vi "MainRunExp.vi"() -> ()   [LabVIEW 2019, in "MotorPID.lvlib"]
uses:
  MotorPID.lvlib
  RunState.ctl
  <vilib>/myRIO/Instrument Drivers/Onboard IO/DIO/typedefs/DIO Reference.ctl
  <vilib>/myRIO/Common/Instrument Driver Framework/Utilities/typedefs/myRIO Generic Hardware Reference.ctl
  <vilib>/myRIO/Common/Instrument Driver Framework/Utilities/typedefs/Hardware Version Enum.ctl
  <vilib>/myRIO/Common/Instrument Driver Framework/Utilities/typedefs/myRIO v1.0 Reference.ctl
  <vilib>/myRIO/Common/Instrument Driver Framework/Utilities/typedefs/Generic FPGA Reference.ctl
  <vilib>/myRIO/Common/Instrument Driver Framework/myRIO v1.0/DIO/typedefs/DIO Channels List.ctl
  <vilib>/myRIO/Common/Instrument Driver Framework/myRIO v1.0/DIO/typedefs/DIO Channels Enum.ctl
  <vilib>/userDefined/High Color/nirio_resource_hc.ctl
  <vilib>/Platform/TimedLoop/XDataNode/timing_clust.ctl
  <vilib>/Platform/TimedLoop/XDataNode/nitl_modes.ctl
  <vilib>/Platform/TimedLoop/XDataNode/wakeup.ctl
  <vilib>/myRIO/Common/Instrument Driver Framework/Utilities/vis/Is FPGA Ref Available.vi
  <vilib>/myRIO/Common/Instrument Driver Framework/ELVIS III v1.0/DIO/vis/ELVIS III v1.1 Open DIO.vi
  <vilib>/myRIO/Instrument Drivers/Onboard IO/DIO/vis/Write.vi
  <vilib>/myRIO/Common/Instrument Driver Framework/Utilities/vis/Validate Channels.vi
  <vilib>/myRIO/Common/Instrument Driver Framework/ELVIS III v1.0/DIO/vis/ELVIS III v1.0 Reserve DIO.vi
  <vilib>/myRIO/Common/Instrument Driver Framework/myRIO v1.0/UART/vis/myRIO v1.0 Close UART.vi
  <vilib>/myRIO/Common/Instrument Driver Framework/ELVIS III v1.0/DIO/vis/ELVIS III v1.0 Build MUX Configuration DIO.vi
  <vilib>/myRIO/Common/Instrument Driver Framework/ELVIS III v1.0/Resource Manager/vis/ELVIS III v1.0 Reserve Channel List.vi
  <vilib>/myRIO/Common/Instrument Driver Framework/ELVIS III v1.0/Resource Manager/vis/ELVIS III v1.0 Create Configuration List.vi
  <vilib>/myRIO/Common/Instrument Driver Framework/ELVIS III v1.0/Resource Manager/vis/ELVIS III v1.0 Reserve Channel.vi
  <vilib>/myRIO/Common/Instrument Driver Framework/ELVIS III v1.0/Resource Manager/vis/ELVIS III v1.0 Unreserve Channel.vi
  <vilib>/myRIO/Common/Instrument Driver Framework/ELVIS III v1.0/Resource Manager/vis/ELVIS III v1.0 Build Mutex Name.vi
  <vilib>/Utility/VariantDataType/GetNumericInfo.vi
  <vilib>/Utility/error.llb/Error Cluster From Error Code.vi
  <vilib>/myRIO/Common/Instrument Driver Framework/ELVIS III v1.0/ELVIS III v1.1 Open.vi
  <vilib>/myRIO/Common/Instrument Driver Framework/Utilities/vis/IO Manager.vi
  <vilib>/myRIO/Common/Instrument Driver Framework/Utilities/vis/Configuration Manager.vi
  <vilib>/myRIO/Common/Instrument Driver Framework/ELVIS III v1.0/Resource Manager/vis/ELVIS III v1.0 Configure IO.vi
  <vilib>/myRIO/Common/Instrument Driver Framework/myRIO v1.0/myRIO v1.0 Close.vi
  <vilib>/myRIO/Common/Instrument Driver Framework/ELVIS III v1.0/DIO/vis/ELVIS III v1.0 Write DIO.vi
  <vilib>/addons/control/pid/pid.llb/PID (DBL).vi
  <vilib>/myRIO/Common/Instrument Driver Framework/Utilities/vis/FPGA Ref Manager.vi
  <vilib>/myRIO/Common/Instrument Driver Framework/ELVIS III v1.0/ELVIS III v1.0 Reset FPGA.vi
  <vilib>/myRIO/Common/Instrument Driver Framework/myRIO v1.0/IRQ/vis/myRIO v1.0 IRQ Info FGV.vi
  <vilib>/myRIO/Common/Instrument Driver Framework/myRIO v1.0/IRQ/vis/myRIO v1.0 Timer IRQ Info FGV.vi
  <vilib>/myRIO/Common/Instrument Driver Framework/myRIO v1.0/IRQ/vis/myRIO v1.0 ISR Agent.vi
  <vilib>/myRIO/Instrument Drivers/Utilities/vis/Reset Index.vi
  <vilib>/myRIO/Common/Instrument Driver Framework/myRIO v1.0/Resource Manager/vis/myRIO v1.0 Block Write Resource Manager.vi
  <vilib>/myRIO/Express VI/Onboard IO/DO/DO Express VI.xnode
  <vilib>/myRIO/Instrument Drivers/Onboard IO/DIO/vis/myRIO DIO Open.xnode
  <vilib>/Platform/TimedLoop/XDataNode/XDataNode.xnode
  <vilib>/Platform/TimedLoop/XDataNode/XDNodeRunTimeDep.lvlib
  <vilib>/myRIO/Instrument Drivers/Onboard IO/DIO/DIO.lvlib
  <vilib>/myRIO/Instrument Drivers/Utilities/Utilities.lvlib
  <vilib>/ptbypt/NI_PtbyPt.lvlib
  <vilib>/addons/control/pid/NI_PID_pid.lvlib
panel:
  out "x >= y?":bool
  out "Boolean":bool
  out "State":u16(ring) items=["StickReset", "MotorReset", "MotorHome", "RunUp", "Runing", "Exit"]
  out "Waveform Chart":T1(graph)
  in  "Setpoint(deg)":dbl(knob) scale=80.0..-80.0
  out "error out":errorcluster
  out "Position(deg)":dbl(knob) scale=80.0..-80.0
  in  "Reset":bool
  in  "Stop Button":bool
  out "MotorResetPOS":dbl[](array[numeric])
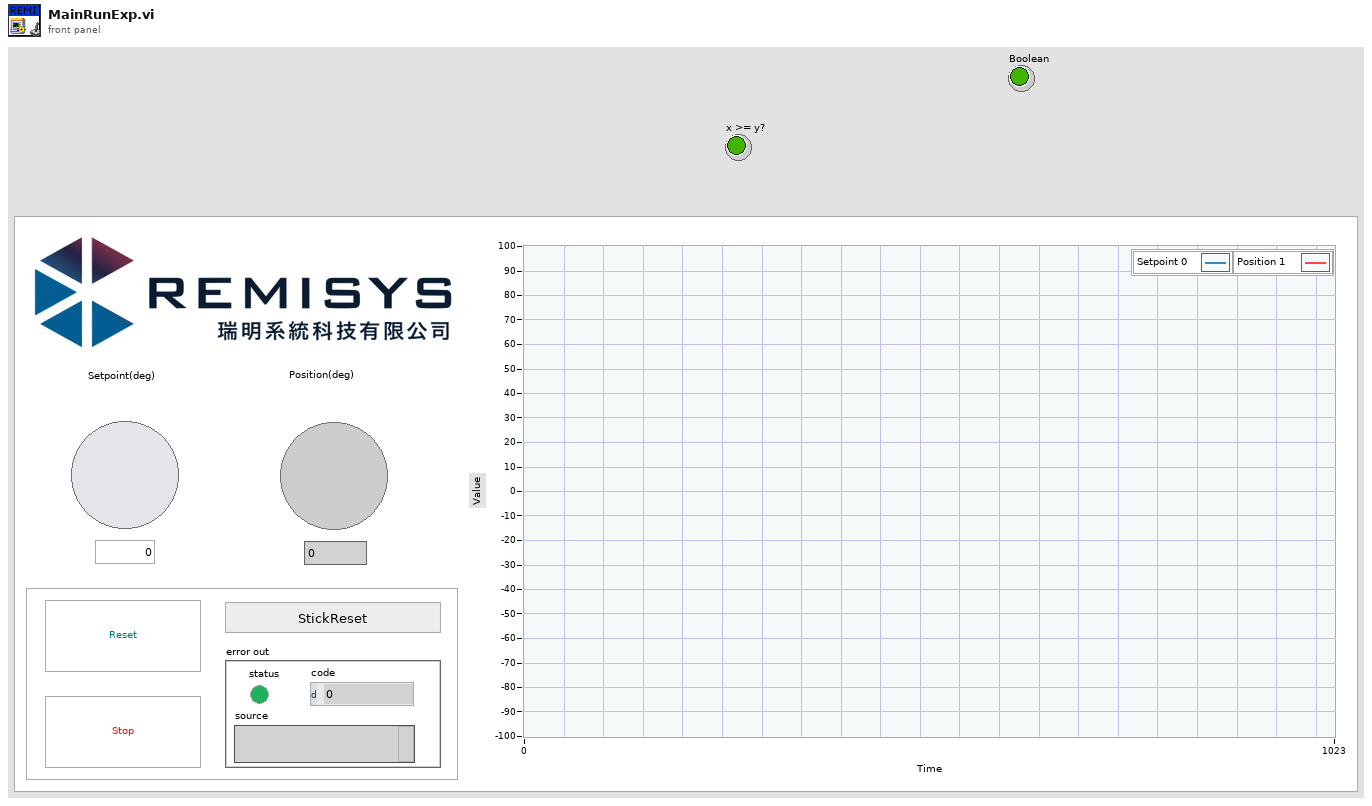
[diagram p1: front panel]
types:
  T1 = cluster{"Setpoint(deg)":dbl, "PresentPOS(deg)":dbl}
  T2 = typedef "MotorPID.lvlib/RunState.ctl" = enum16{"StickReset", "MotorReset", "MotorHome", "RunUp", "Runing", "Exit"}
  T3 = typedef "DIO.lvlib/DIO Reference.ctl" = cluster{"myRIO Reference":T4, "DIO Channels List":T8}
  T4 = typedef "myRIO Generic Hardware Reference.ctl" = cluster{"myRIO Model":T5, "myRIO Hardware Reference":T6}
  T5 = typedef "Hardware Version Enum.ctl" = enum16{"Unknown", "myRIO-1900", "myRIO-1950", "roboRIO", "NI ELVIS RIO CM", "ELVIS III"}
  T6 = typedef "myRIO v1.0 Reference.ctl" = cluster{"Generic FPGA Reference":T7, "Allow multiple opens":bool}
  T7 = typedef "Generic FPGA Reference.ctl" = refnum<k20>
  T8 = typedef "DIO Channels List.ctl" = T9[]
  T9 = typedef "DIO Channels Enum.ctl" = enum16{"Not Connected", "C/DIO0", "C/DIO1", "C/DIO2", "C/DIO3", "C/DIO4", "C/DIO5", "C/DIO6", "C/DIO7", "A/DIO0", "A/DIO1", "A/DIO2", "A/DIO3", "A/DIO4", "A/DIO5", "A/DIO6", "A/DIO7", "A/DIO8", "A/DIO9", "A/DIO10", "A/DIO11", "A/DIO12", "A/DIO13", "A/DIO14", "A/DIO15", "A/DIO16", "A/DIO17", "A/DIO18", "A/DIO19", "B/DIO0", "B/DIO1", "B/DIO2", "B/DIO3", "B/DIO4", "B/DIO5", "B/DIO6", "B/DIO7", "B/DIO8", "B/DIO9", "B/DIO10", "B/DIO11", "B/DIO12", "B/DIO13", "B/DIO14", "B/DIO15", "B/DIO16", "B/DIO17", "B/DIO18", "B/DIO19", "LED0", "LED1", "LED2", "LED3", "Button0", "DIO/DIO0", "DIO/DIO1", "DIO/DIO2", "DIO/DIO3", "DIO/DIO4", "DIO/DIO5", "DIO/DIO6", "DIO/DIO7", "DIO/DIO8", "DIO/DIO9", "SPI/CS0", "SPI/CS1", "SPI/CS2", "SPI/CS3", "LED RADIO (Green)", "LED RADIO (Red)", "LED COMM (Green)", "LED COMM (Red)", "LED MODE (Green)", "LED MODE (Red)"}
  T10 = typedef "nirio_resource_hc.ctl" = tag
  T11 = typedef "XDNodeRunTimeDep.lvlib/timing_clust.ctl" = cluster{"Expected End [f-1]":u64, "Actual End [f-1]":u64, "Finished Late? [f-1]":bool, "Expected End [i-1]":u64, "Actual End [i-1]":u64, "Finished Late? [i-1]":bool, "Expected Start [i]":u64, "Actual Start [i]":u64, "Expected Start [f]":u64, "Actual Start [f]":u64, "Source Name":string, "Structure Name":string, "Period":i64, "Deadline":i64, "Offset":i64, "Start":i64, "Priority":i32, "Timeout":i32, "Mode":T12, "Wakeup Reason":T13, "Error":errorcluster, "Source Type":string, "Secondary Source Type":string, "Global End Time":u64, "Global Start Time":u64, "Frame Duration":u64, "Iteration Duration":u64, "Assigned CPU":i32, "I/O Scan Engine Mode":u32}
  T12 = typedef "XDNodeRunTimeDep.lvlib/nitl_modes.ctl" = enum32{"No Change", "Process missed periods, maintain original phase", "Discard missed periods, maintain original phase", "Process missed periods, ignore original phase", "Discard missed periods, ignore original phase"}
  T13 = typedef "XDNodeRunTimeDep.lvlib/wakeup.ctl" = enum32{"Normal", "Aborted", "Asynchronous wakeup", "Timing source error", "Timed loop error", "Timeout"}
  T14 = cluster{"proportional gain (Kc)":dbl, "integral time (Ti, min)":dbl, "derivative time (Td, min)":dbl}
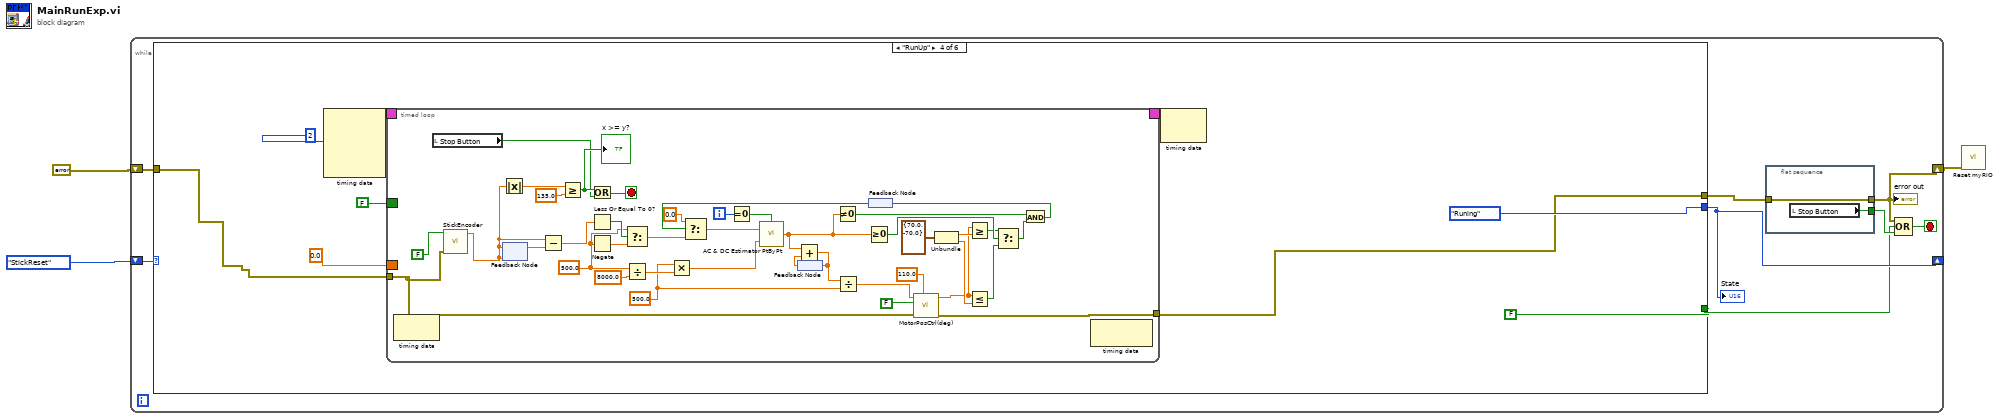
[diagram p0: block diagram]
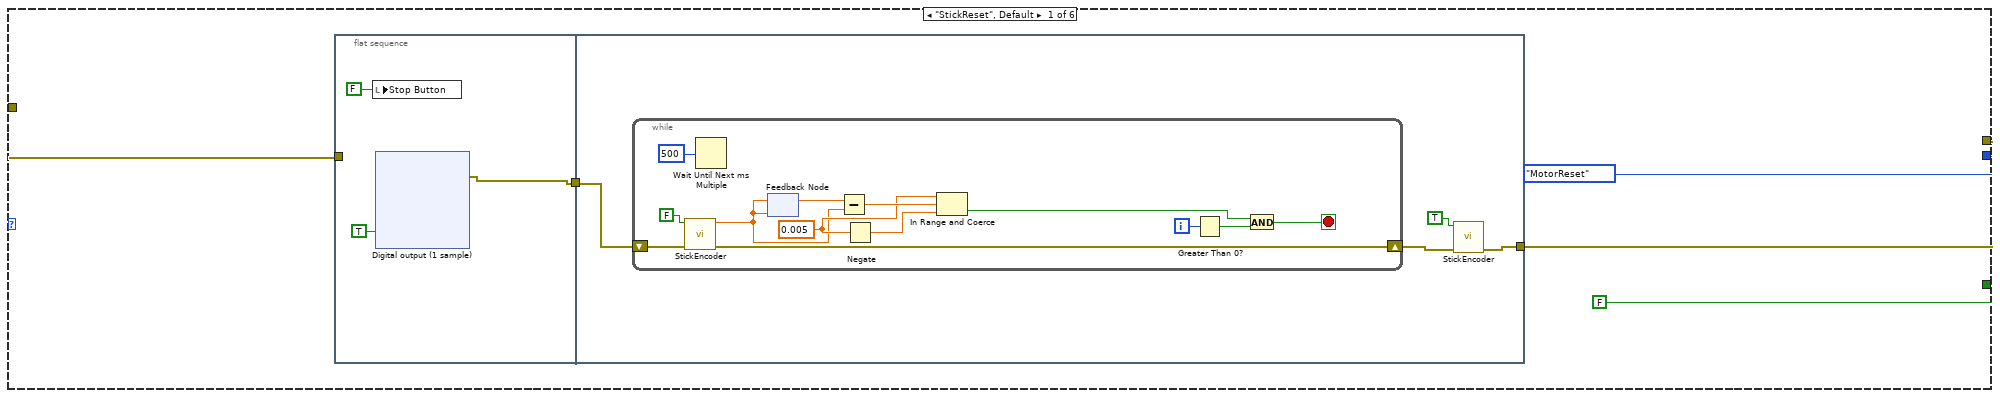
[diagram p2: hidden frame]
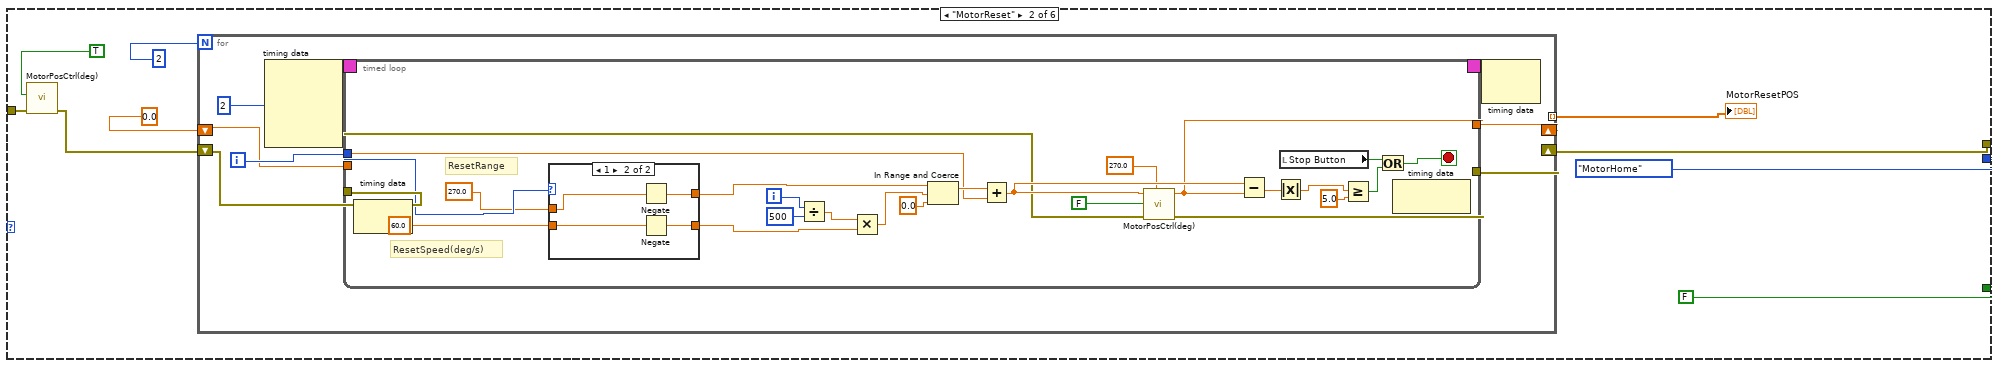
[diagram p3: hidden frame]
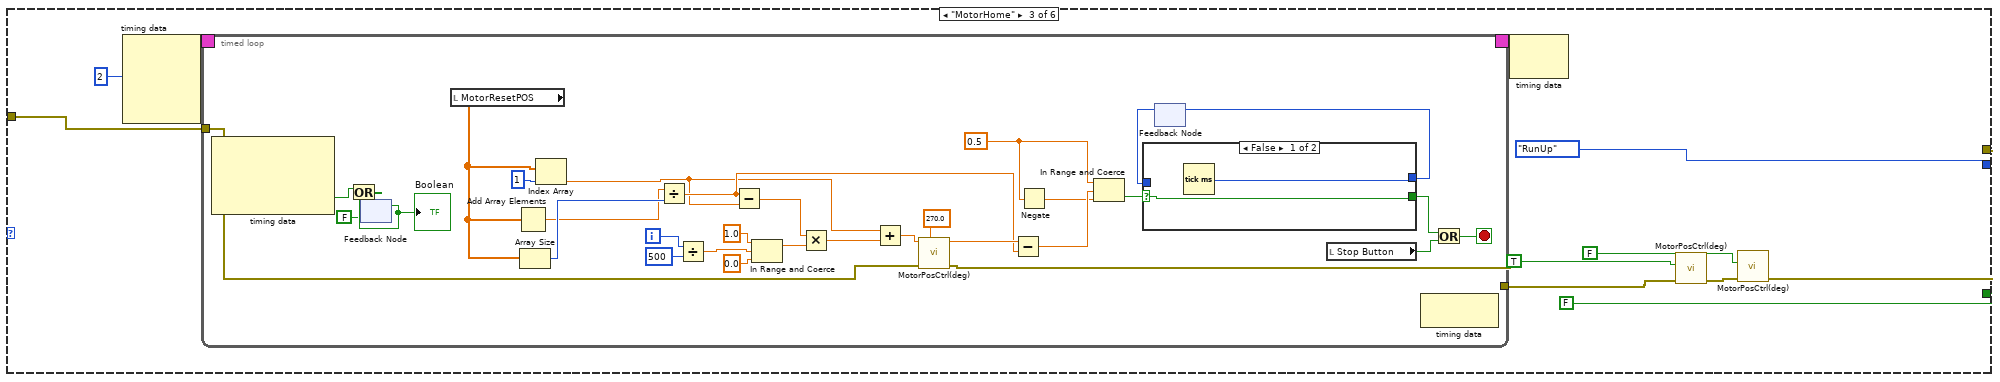
[diagram p5: hidden frame]
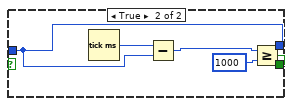
[diagram p6: hidden frame]
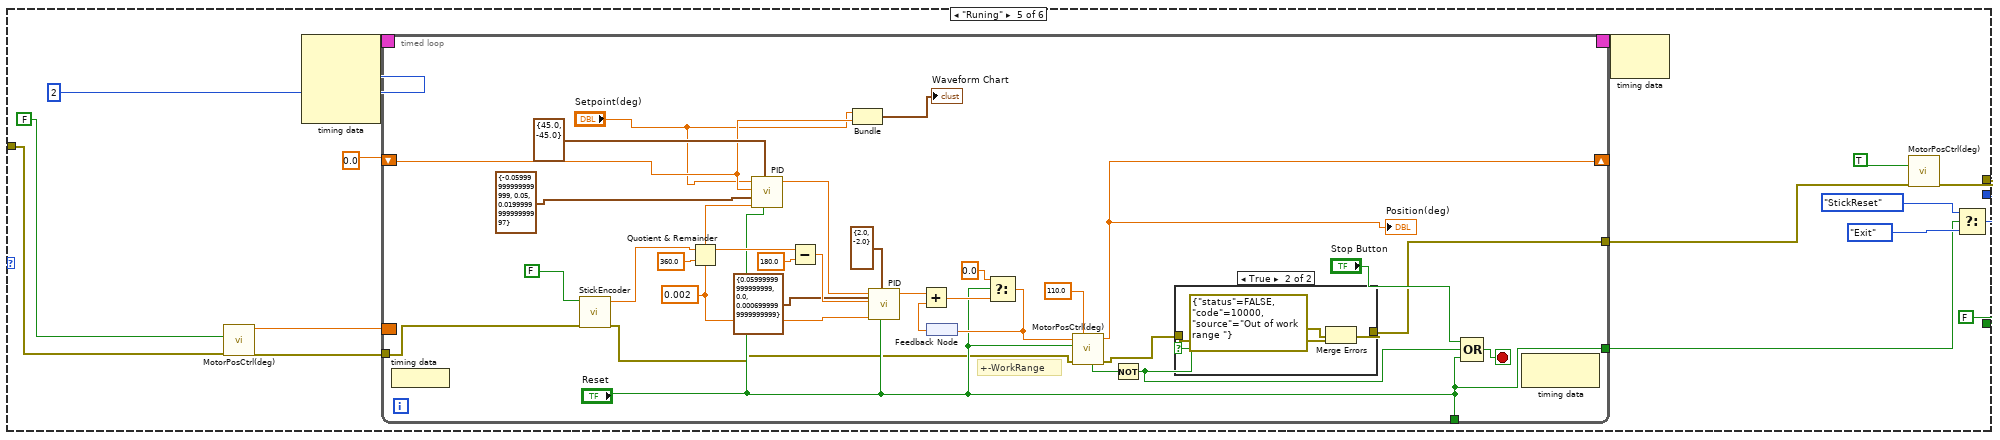
[diagram p7: hidden frame]
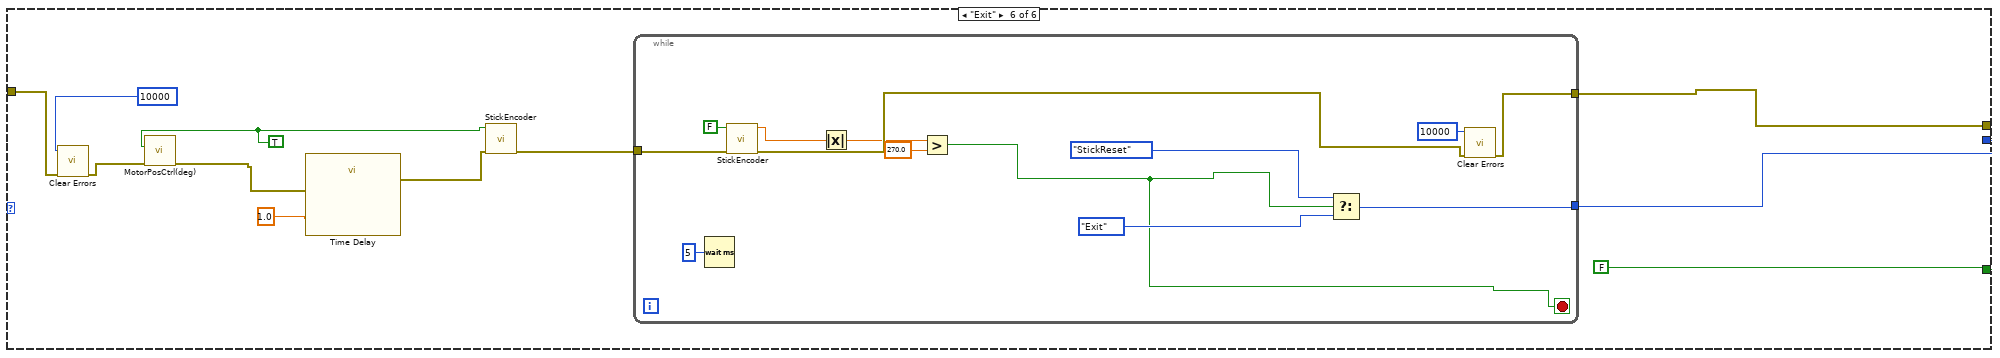
[diagram p9: hidden frame]
diagram:
  n1 = while {
    shift-right: [w6] -> _
    shift-left: RunState."StickReset" -> [w11]
    shift-right: [w5] -> w1
    shift-left: errorcluster {"status"=FALSE, "code"=0, "source"=""} ("error in (no error)") -> [w10]
    stop <- w9 stop-if-true
    n2 = case shown="\"RunUp\"" w11 {
      tunnel: w10 -> [w16 w76 w134 w185 w254 w303]
      tunnel: [w17 w82 w128 w184 w251 w301] -> w8
      tunnel: [RunState."MotorReset" RunState."MotorHome" RunState."RunUp" RunState."Runing" w248 w305] -> w6
      tunnel: [FALSE FALSE FALSE FALSE FALSE FALSE] -> w4
      frame "StickReset", Default {
        n3 = flat-sequence {
          tunnel: w16 -> [_]
          tunnel: [w19] -> w15
          tunnel: [w58] -> w17
          tunnel: w15 -> [w57]
          frame #0 {
            n4 = local write "Stop Button"(FALSE ("Stop Button")) -> ()
            n5 = xnode "Digital output (1 sample)"("ENA (A/DIO5)"=TRUE) -> ("error out"=w19:errorcluster)  [unwired: 1 in]
          }
          frame #1 {
            n6 = while {
              shift-right: [w73] -> w60
              shift-left: w57 -> [w72]
              i -> [w66]
              stop <- w63 stop-if-true
              w68 = 0.005 ("upper limit")
              n7 = call "StickEncoder.vi"("error in (no error)"=w72, "Reset Counter"=FALSE) -> ("error out"=w73:errorcluster, "PresentPOS(deg)"=w61:dbl)  [unwired: 8 in]
              n8 = Wait Until Next ms Multiple(millisecond multiple=u32 500) -> ()  [unwired: 1 out]
              n9 = feedback-in #1(w61) -> ()
              n10 = feedback #1(w61) -> (w70:dbl)
              n11 = Subtract(x=w70, y=w61) -> (x-y=w69:dbl)
              n12 = Negate(x=w68) -> (-x=w67:dbl)
              n13 = In Range and Coerce(upper limit=w68, x=w69, lower limit=w67) -> (In Range?=w65:bool)  [unwired: 1 out]
              n14 = Greater Than 0?(x=w66) -> (x > 0?=w64:bool)
              n15 = And(x=w65, y=w64) -> (x .and. y?=w63:bool)
            }
            n16 = call "StickEncoder.vi"("error in (no error)"=w60, "Reset Counter"=TRUE) -> ("error out"=w58:errorcluster)  [unwired: 8 in, 1 out]
          }
        }
      }
      frame "MotorReset" {
        n17 = call "MotorPosCtrl(deg).vi"("error in (no error)"=w76, "Reset Button"=TRUE) -> ("error out"=w77:errorcluster)  [unwired: 6 in, 3 out]
        n18 = for {
          N: 2 -> [_]
          shift-right: [w87] -> w82
          shift-left: w77 -> [w86]
          shift-right: [w83] -> _
          shift-left: 0.0 ("PresentPOS(deg)") -> [w84]
          tunnel: [w83] -> w79 mode=indexing
          i -> [w85]
          n19 = node-c288(i64 2 ("Period")) -> (w90:T11)  [unwired: 3 in]
          n20 = timed-loop {
            timing: w90 -> [_]
            timing-out: [_] -> w89
            tunnel: w86 -> [w91]
            tunnel: [w114] -> w87
            tunnel: w85 -> [w109]
            tunnel: [w97] -> w83
            tunnel: w84 -> [w106]
            i -> [w113]
            stop <- w101 stop-if-true
            # "ResetRange"
            # "ResetSpeed(deg/s)"
            n21 = node-c288() -> ()  [unwired: 1 in, 1 out]
            n22 = case shown="1" w109 {
              tunnel: [w116 w119] -> w108
              tunnel: [w115 w117] -> w104
              tunnel: 270.0 ("Target(deg)") -> [w116 w120]
              tunnel: 60.0 ("y") -> [w115 w118]
              frame 0, Default {
              }
              frame 1 {
                n23 = Negate(x=w120) -> (-x=w119:dbl)
                n24 = Negate(x=w118) -> (-x=w117:dbl)
              }
            }
            n25 = Divide(x=w113, y=500) -> (x/y=w112:dbl)
            n26 = Multiply(x=w112, y=w104) -> (x*y=w111:dbl)
            n27 = In Range and Coerce(upper limit=w108, x=w111, lower limit=0.0) -> (coerced(x)=w107:dbl)  [unwired: 1 out]
            n28 = Add(x=w107, y=w106) -> (x+y=w98:dbl)
            n29 = call "MotorPosCtrl(deg).vi"("WorkRange 2"=270.0 ("WorkRange"), "error in (no error)"=w91, "Reset Button"=FALSE, "Target(deg)"=w98) -> ("error out"=w114:errorcluster, "PresentPOS(deg)"=w97:dbl)  [unwired: 4 in, 2 out]
            n30 = Subtract(x=w98, y=w97) -> (x-y=w95:dbl)
            n31 = Absolute Value(x=w95) -> (abs(x)=w94:dbl)
            n32 = local read "Stop Button"() -> (w100:bool)
            n33 = Greater Or Equal?(x=w94, y=5.0) -> (x >= y?=w93:bool)
            n34 = Or(x=w100, y=w93) -> (x .or. y?=w101:bool)
            n35 = node-c288() -> ()  [unwired: 1 in, 1 out]
          }
          n36 = node-c288(w89) -> ()  [unwired: 1 out]
        }
        "MotorResetPOS" <- w79
      }
      frame "MotorHome" {
        n37 = node-c288(i64 2 ("Period")) -> (w136:T11)  [unwired: 3 in]
        n38 = timed-loop {
          timing: w136 -> [_]
          timing-out: [_] -> w135
          tunnel: w134 -> [w169]
          tunnel: [w163] -> w132
          i -> [w157]
          stop <- w143 stop-if-true
          w165 = 0.5
          n39 = node-c288() -> (w141:bool)  [unwired: 1 in, 3 out]
          n40 = feedback #2(FALSE) -> (w139:bool)
          "Boolean" <- w139
          n41 = Or(x=w141, y=w139) -> (x .or. y?=w140:bool)
          n42 = feedback-in #2(w140) -> ()
          n43 = local read "MotorResetPOS"() -> (w152:dbl[])
          n44 = Add Array Elements(numeric array=w152) -> (sum=w151:dbl)
          n45 = Array Size(array=w152) -> (size(s)=w168:i32)
          n46 = Index Array(array=w152, index=1) -> (element=w146:dbl)
          n47 = Divide(x=w151, y=w168) -> (x/y=w148:dbl)
          n48 = Divide(x=w157, y=500) -> (x/y=w155:dbl)
          n49 = Subtract(x=w148, y=w146) -> (x-y=w147:dbl)
          n50 = In Range and Coerce(upper limit=1.0, x=w155, lower limit=0.0) -> (coerced(x)=w150:dbl)  [unwired: 1 out]
          n51 = Multiply(x=w147, y=w150) -> (x*y=w149:dbl)
          n52 = Add(x=w146, y=w149) -> (x+y=w145:dbl)
          n53 = call "MotorPosCtrl(deg).vi"("WorkRange 2"=270.0 ("WorkRange"), "error in (no error)"=w169, "Target(deg)"=w145) -> ("error out"=w163:errorcluster, "PresentPOS(deg)"=w167:dbl)  [unwired: 5 in, 2 out]
          n54 = Subtract(x=w167, y=w148) -> (x-y=w166:dbl)
          n55 = Negate(x=w165) -> (-x=w164:dbl)
          n56 = In Range and Coerce(upper limit=w165, x=w166, lower limit=w164) -> (In Range?=w158:bool)  [unwired: 1 out]
          n57 = feedback #3() -> (w161:u32)  [unwired: 1 in]
          n58 = case shown="False" w158 {
            selector: w158 -> [w170 _]
            tunnel: [w171 w172] -> w162
            tunnel: w161 -> [_ w172]
            tunnel: [w170 w173] -> w159
            frame False {
              n59 = Tick Count (ms)() -> (millisecond timer value=w171:u32)
            }
            frame True {
              n60 = Tick Count (ms)() -> (millisecond timer value=w176:u32)
              n61 = Subtract(x=w176, y=w172) -> (x-y=w175:u32)
              n62 = Greater Or Equal?(x=w175, y=u32 1000) -> (x >= y?=w173:bool)
            }
          }
          n63 = feedback-in #3(w162) -> ()
          n64 = local read "Stop Button"() -> (w160:bool)
          n65 = node-c288() -> ()  [unwired: 1 in, 1 out]
          n66 = Or(x=w159, y=w160) -> (x .or. y?=w143:bool)
        }
        n67 = node-c288(w135) -> ()  [unwired: 1 out]
        n68 = call "MotorPosCtrl(deg).vi"("error in (no error)"=w132, "Reset Button"=TRUE) -> ("error out"=w129:errorcluster)  [unwired: 6 in, 3 out]
        n69 = call "MotorPosCtrl(deg).vi"("error in (no error)"=w129, "Reset Button"=FALSE) -> ("error out"=w128:errorcluster)  [unwired: 6 in, 3 out]
      }
      frame "RunUp" {
        n70 = node-c288(i64 2 ("Period")) -> (w190:T11)  [unwired: 3 in]
        n71 = timed-loop {
          timing: w190 -> [_]
          timing-out: [_] -> w189
          tunnel: w185 -> [w198]
          tunnel: [w193] -> w184
          border: 0.0 ("PresentPOS(deg)") -> [_]
          border: FALSE -> [_]
          i -> [w232]
          stop <- w226 stop-if-true
          w222 = 500.0 ("MaxSpeed(deg/s)")
          w212 = 500.0 ("x")
          n72 = node-c288() -> ()  [unwired: 1 in, 1 out]
          n73 = local read "Stop Button"() -> (w199:bool)
          n74 = call "StickEncoder.vi"("error in (no error)"=w198, "Reset Counter"=FALSE) -> ("PresentPOS(deg)"=w201:dbl)  [unwired: 8 in, 1 out]
          n75 = Absolute Value(x=w201) -> (abs(x)=w229:dbl)
          n76 = feedback-in #4(w201) -> ()
          n77 = feedback #4(w201) -> (w230:dbl)
          n78 = Subtract(x=w201, y=w230) -> (x-y=w225:dbl)
          n79 = Greater Or Equal?(x=w229, y=135.0) -> (x >= y?=w227:bool)
          "x >= y?" <- w227
          n80 = Or(x=w227, y=w199) -> (x .or. y?=w226:bool)
          n81 = Less Or Equal To 0?(x=w225) -> (x <= 0?=w224:bool)
          n82 = Negate(x=w222) -> (-x=w223:dbl)
          n83 = Select(t=w222, s=w224, f=w223) -> (s? t:f=w216:dbl)
          n84 = Divide(x=w222, y=8000.0 ("Acc(deg/ss)")) -> (x/y=w221:dbl)
          n85 = Multiply(x=w212, y=w221) -> (x*y=w202:dbl)
          n86 = Equal To 0?(x=w232) -> (x = 0?=w231:bool)
          n87 = feedback #5() -> (w219:dbl)
          n88 = feedback #6() -> (w217:bool)
          n89 = Select(t=0.0, s=w217, f=w216) -> (s? t:f=w214:dbl)
          n90 = call <vilib>:"AC & DC Estimator PtByPt.vi"("signal"=w214, "sample length"=w202, "initialize"=w231) -> ("DC estimate (V)"=w206:dbl)  [unwired: 2 out]
          n91 = Add(x=w206, y=w219) -> (x+y=w213:dbl)
          n92 = feedback-in #5(w213) -> ()
          n93 = Not Equal To 0?(x=w206) -> (x != 0?=w205:bool)
          n94 = Divide(x=w213, y=w212) -> (x/y=w196:dbl)
          n95 = Greater Or Equal To 0?(x=w206) -> (x >= 0?=w211:bool)
          n96 = call "MotorPosCtrl(deg).vi"("WorkRange 2"=110.0 ("WorkRange"), "error in (no error)"=w198, "Reset Button"=FALSE, "Target(deg)"=w196) -> ("error out"=w193:errorcluster, "PresentPOS(deg)"=w194:dbl)  [unwired: 4 in, 2 out]
          n97 = Unbundle(cluster{"UpLimit":dbl, "DownLimit":dbl} {"UpLimit"=70.0, "DownLimit"=-70.0} ("RunUpLimuit")) -> ("UpLimit"=w210:dbl, "DownLimit"=w209:dbl)
          n98 = Greater Or Equal?(x=w194, y=w210) -> (x >= y?=w208:bool)
          n99 = Less Or Equal?(x=w194, y=w209) -> (x <= y?=w207:bool)
          n100 = Select(t=w208, s=w211, f=w207) -> (s? t:f=w204:bool)
          n101 = And(x=w205, y=w204) -> (x .and. y?=w203:bool)
          n102 = feedback-in #6(w203) -> ()
          n103 = node-c288() -> ()  [unwired: 1 in, 1 out]
        }
        n104 = node-c288(w189) -> ()  [unwired: 1 out]
      }
      frame "Runing" {
        n105 = call "MotorPosCtrl(deg).vi"("error in (no error)"=w254, "Reset Button"=FALSE) -> ("error out"=w242:errorcluster, "PresentPOS(deg)"=w241:dbl)  [unwired: 6 in, 2 out]
        n106 = node-c288(i64 2 ("Period")) -> (w246:T11)  [unwired: 3 in]
        n107 = timed-loop "Timed Loop" {
          timing: w246 -> [_]
          timing-out: [_] -> w245
          border: w241 -> [_]
          shift-right: [w270] -> _
          shift-left: 0.0 -> [w272]
          tunnel: w242 -> [w259]
          tunnel: ["Reset"] -> _
          tunnel: ["Reset"] -> w240
          tunnel: [w255] -> w239
          stop <- w273 stop-if-true
          w281 = 0.002 ("dt (s)")
          # "+-WorkRange"
          n108 = node-c288() -> ()  [unwired: 1 in]
          n109 = call "StickEncoder.vi"("error in (no error)"=w259, "Reset Counter"=FALSE) -> ("error out"=w261:errorcluster, "PresentPOS(deg)"=w262:dbl)  [unwired: 8 in]
          n110 = Quotient & Remainder(x=w262, y=360.0) -> (x-y*floor(x/y)=w274:dbl)  [unwired: 1 out]
          n111 = call-poly <vilib>:"PID.vi"("reinitialize? (F)"="Reset", "output range"=cluster{"output high":dbl, "output low":dbl} {"output high"=45.0, "output low"=-45.0}, "dt (s)"=w281, "PID gains"=T14 {"proportional gain (Kc)"=-0.05999999999999999, "integral time (Ti, min)"=0.05, "derivative time (Td, min)"=0.019999999999999997} ("PID gains 2"), "process variable"=w272, "setpoint"="Setpoint(deg)") -> ("output"=w276:dbl)  [unwired: 4 in, 1 out]
          n112 = Subtract(x=w274, y=180.0) -> (x-y=w280:dbl)
          n113 = Bundle("Setpoint(deg)"="Setpoint(deg)", w272) -> (→"Waveform Chart":cluster{"Setpoint(deg)":dbl, dbl})  [unwired: 1 in]
          n114 = call-poly <vilib>:"PID.vi"("reinitialize? (F)"="Reset", "output range"=cluster{"output high":dbl, "output low":dbl} {"output high"=2.0, "output low"=-2.0}, "dt (s)"=w281, "PID gains"=T14 {"proportional gain (Kc)"=0.05999999999999999, "integral time (Ti, min)"=0.0, "derivative time (Td, min)"=0.0006999999999999999}, "process variable"=w280, "setpoint"=w276) -> ("output"=w278:dbl)  [unwired: 4 in, 1 out]
          n115 = feedback #7() -> (w284:dbl)
          n116 = Add(x=w278, y=w284) -> (x+y=w283:dbl)
          n117 = Select(t=0.0, s="Reset", f=w283) -> (s? t:f=w264:dbl)
          n118 = feedback-in #7(w264) -> ()
          n119 = call "MotorPosCtrl(deg).vi"("WorkRange 2"=110.0 ("WorkRange"), "error in (no error)"=w261, "Reset Button"="Reset", "Target(deg)"=w264) -> ("error out"=w266:errorcluster, "PresentPOS(deg)"=w270:dbl, "In Range?"=w267:bool)  [unwired: 4 in, 1 out]
          "Position(deg)" <- w270
          n120 = Not(x=w267) -> (.not. x?=w256:bool)
          n121 = case shown="True" w256 {
            tunnel: w266 -> [w286 w289]
            tunnel: [w286 w287] -> w255
            frame False {
            }
            frame True {
              n122 = Merge Errors(errorcluster {"status"=FALSE, "code"=10000, "source"="Out of work range "} ("error in (no error)"), w289) -> (w287:errorcluster)
            }
          }
          n123 = Compound Arithmetic op=OR("Stop Button", w256, "Reset") -> (w273:bool)
          n124 = node-c288() -> ()  [unwired: 1 in, 1 out]
        }
        n125 = node-c288(w245) -> ()  [unwired: 1 out]
        n126 = call "MotorPosCtrl(deg).vi"("error in (no error)"=w239, "Reset Button"=TRUE) -> ("error out"=w251:errorcluster)  [unwired: 6 in, 3 out]
        n127 = Select(t=RunState."StickReset", s=w240, f=RunState."Exit") -> (s? t:f=w248:T2)
      }
      frame "Exit" {
        w298 = TRUE ("Reset Counter")
        n128 = call <vilib>:"Clear Errors.vi"("error in (no error)"=w303, "specific error code to clear (0: all)"=10000) -> ("error out"=w300:errorcluster)  [unwired: 4 in, 1 out]
        n129 = call "MotorPosCtrl(deg).vi"("error in (no error)"=w300, "Reset Button"=w298) -> ("error out"=w299:errorcluster)  [unwired: 6 in, 3 out]
        n130 = call "Time Delay"("error in (no error)"=w299, "Delay Time (s)"=1.0) -> ("error out"=w297:errorcluster)  [unwired: 9 in]
        n131 = call "StickEncoder.vi"("error in (no error)"=w297, "Reset Counter"=w298) -> ("error out"=w296:errorcluster)  [unwired: 8 in, 1 out]
        n132 = while {
          tunnel: w296 -> [w319]
          tunnel: [w313] -> w305
          tunnel: [w309] -> w301
          stop <- w308 stop-if-true
          n133 = Wait (ms)(milliseconds to wait=u32 5) -> ()  [unwired: 1 out]
          n134 = call "StickEncoder.vi"("error in (no error)"=w319, "Reset Counter"=FALSE) -> ("error out"=w310:errorcluster, "PresentPOS(deg)"=w316:dbl)  [unwired: 8 in]
          n135 = Absolute Value(x=w316) -> (abs(x)=w307:dbl)
          n136 = Greater?(x=w307, y=270.0) -> (0:w308:bool)
          n137 = Select(t=RunState."StickReset", s=w308, f=RunState."Exit") -> (s? t:f=w313:T2)
          n138 = call <vilib>:"Clear Errors.vi"("error in (no error)"=w310, "specific error code to clear (0: all)"=10000) -> ("error out"=w309:errorcluster)  [unwired: 4 in, 1 out]
        }
      }
    }
    "State" <- w6
    n139 = flat-sequence {
      tunnel: w8 -> [w12]
      tunnel: [w13] -> w7
      tunnel: [w12] -> w5
      frame #0 {
        n140 = local read "Stop Button"() -> (w13:bool)
      }
    }
    n141 = Compound Arithmetic op=OR(w5, w4, w7) -> (w9:bool)
    "error out" <- w5
  }
  n142 = call <vilib>:"Reset myRIO.vi"("error in (no error)"=w1) -> ()  [unwired: 10 in, 1 out]
